vi "Get id of last record.vi"(8 "error in (no error)":errorcluster, 9 "Alarm Type":string, 10 "table":string, 11 "connection reference":T1) -> (0 "error out":errorcluster, 2 "id":i32, 3 "connection reference 2":T1)   [LabVIEW 2018]
uses:
  <vilib>/addons/database/Connection.llb/Conn ObjectReference.ctl
  <vilib>/addons/database/Connection.llb/Conn Execute.vi
  <vilib>/addons/database/Recordset.llb/Rec Fetch Integer Data (R).vi
  <vilib>/addons/database/Recordset.llb/Rec Destroy - Connection.vi
  <vilib>/addons/database/NI_Database_API.lvlib
panel:
  in  "concatenated string":string
  in  "table 2":string
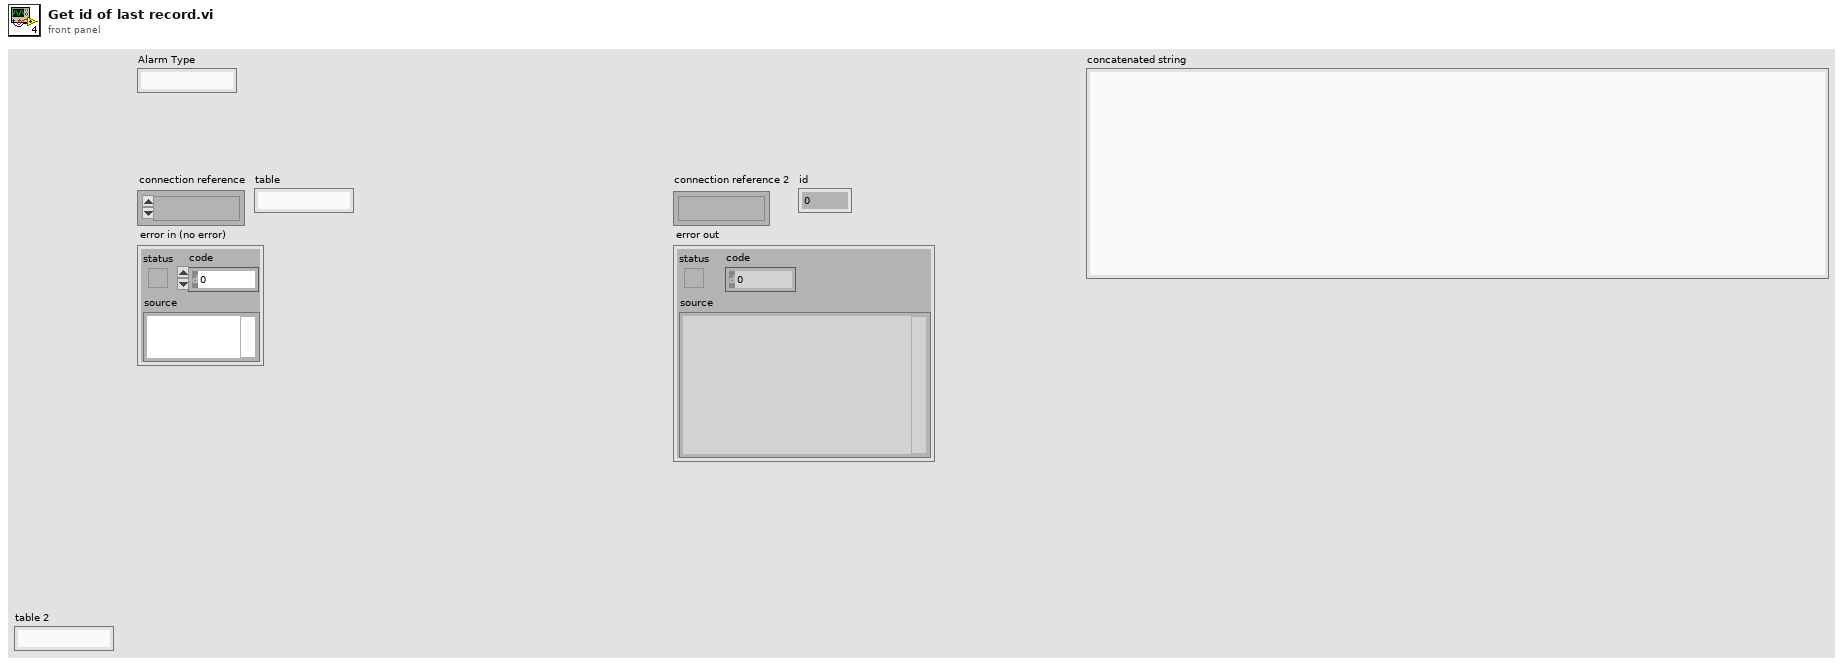
[diagram p1: front panel]
types:
  T1 = typedef "NI_Database_API.lvlib/Conn ObjectReference.ctl" = refnum<k1>
  T2 = typedef "NI_Database_API.lvlib/Rec ObjectReference.ctl" = refnum<k1>
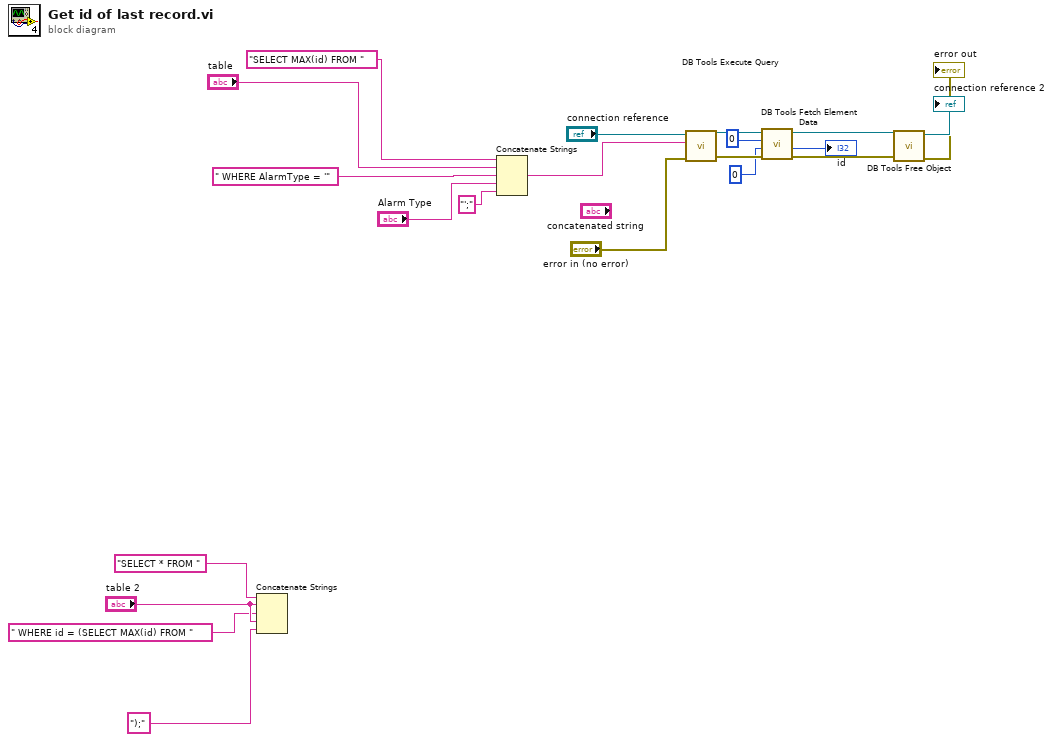
[diagram p0: block diagram]
diagram:
  n1 = Concatenate Strings("SELECT * FROM " ("SQL query"), "table 2", " WHERE id = (SELECT MAX(id) FROM " ("SQL query"), "table 2", ");" ("Substring")) -> ()  [unwired: 1 out]
  n2 = Concatenate Strings("SELECT MAX(id) FROM " ("SQL query"), "table", " WHERE AlarmType = '" ("SQL query"), "Alarm Type", "';" ("string")) -> (w1:string)
  n3 = call-poly <vilib>:"DB Tools Execute Query.vi"("error in (no error)"="error in (no error)", "SQL query"=w1, "connection reference"="connection reference") -> ("error out"=w14:errorcluster, "recordset reference"=w17:T2)  [unwired: 5 in]
  n4 = call-poly <vilib>:"DB Tools Fetch Element Data.vi"("error in (no error)"=w14, "type"=0, "column index"=0, "recordset reference"=w17) -> ("error out"=w15:errorcluster, "data"=→"id":i32, "recordset reference out"=w16:T2)  [unwired: 3 in]
  n5 = call-poly <vilib>:"DB Tools Free Object.vi"("error in (no error)"=w15, "recordset reference"=w16) -> ("error out"=→"error out":errorcluster, "connection reference"=→"connection reference 2":T1)  [unwired: 8 in]
